vi "SetWindowKeyboardGrab.vi"(8 "No Error":errorcluster, 10 "Grabbed":bool, 11 "Window [SDL_Window *]":i64 format="%.0x") -> (0 "Error Out":errorcluster)   [LabVIEW 2024, in "SDL3.lvlib" / "Video.lvlib"]
doc: "<B>Summary</B>\nSet a window's keyboard grab mode.\n\n<B>Remarks</B>\nKeyboard grab enables capture of system keyboard shortcuts like Alt+Tab or the Meta/Super key. Note that not all system keyboard shortcuts can be captured by applications (one example is Ctrl+Alt+Del on Windows).\n\nThis is primarily intended for specialized applications such as VNC clients or VM frontends. Normal games should not use keyboard grab.\n\nWhen keyboard grab is enabled, SDL will continue to handle Alt+Tab when the window is full-screen to ensure the user is not trapped in your application. If you have a custom keyboard shortcut to exit fullscreen mode, you may suppress this behavior with <B>SDL_HINT_ALLOW_ALT_TAB_WHILE_GRABBED</B>.\n\nIf the caller enables a grab while another window is currently grabbed, the other window loses its grab in favor of the caller's window."
uses:
  Video.lvlib
  Lib/SDL3.dll
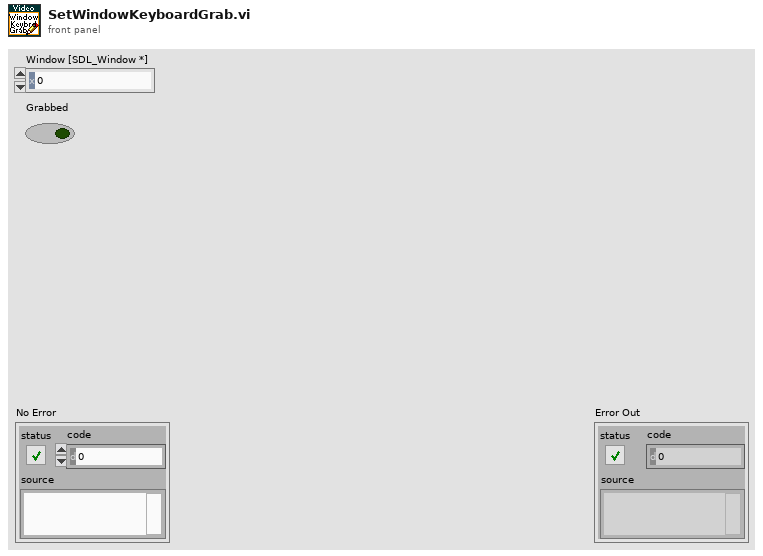
[diagram p1: front panel]
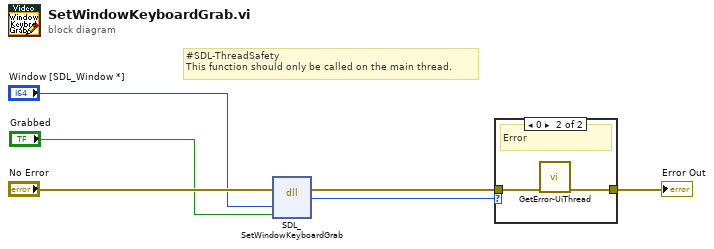
[diagram p0: block diagram]
diagram:
  # "#SDL-ThreadSafety\nThis function should only be called on the main thread."
  n1 = dll-call lib="C:/Users/Thomas/Documents/Projects/LV-SDL3/Sources/SDL3/Lib/SDL3.*" fn="SDL_SetWindowKeyboardGrab"(error in="No Error", "window"="Window [SDL_Window *]", "grabbed"="Grabbed") -> (error out=w3:errorcluster, "return type"=w2:i32)  [unwired: 4 in, 1 out]
  n2 = case shown="0" w2 {
    tunnel: w3 -> [w7 w9]
    tunnel: [w7 w8] -> w5
    frame Default {
      # "Ok"
    }
    frame 0 {
      # "Error"
      n3 = call "GetError-UiThread.vi"("No Error"=w9) -> ("error out"=w8:errorcluster)  [unwired: 10 in]
    }
  }
  "Error Out" <- w5
